vi "TDMS Initialization VI.vi"(8 "error in (no error)":errorcluster, 10 "Custom XML":string, 11 "Device Item Ref in":T1 format="%.0x") -> (0 "error out":errorcluster, 3 "Device Item Ref out":T1 format="%.0x")   [LabVIEW 2011, in "TDMS Custom Device.lvlib"]
uses:
  TDMS Custom Device.lvlib
  <vilib>/NI Veristand/Custom Device API/Custom Device Item Ref.ctl
  <vilib>/NI Veristand/Custom Device API/Custom Device Channel.ctl
  <vilib>/NI Veristand/Custom Device API/Custom Device Channel Type.ctl
  <vilib>/NI Veristand/Custom Device API/Custom Device API.lvlib
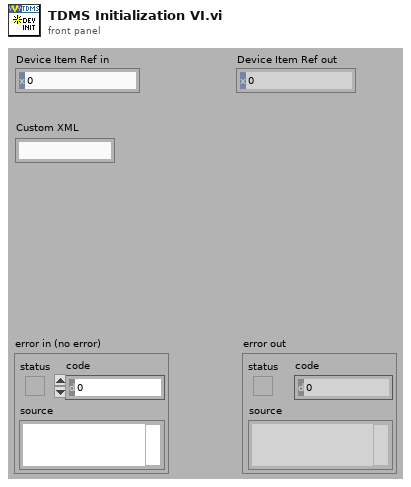
[diagram p1: front panel]
types:
  T1 = typedef "Custom Device API.lvlib/Custom Device Item Ref.ctl" = u64
  T2 = enum16{"Play and Repeat Last", "Stop (and Reset)", "Loop", "Pause"}
  T3 = typedef "Custom Device API.lvlib/Custom Device Channel.ctl" = cluster{"Type":T4, "Units":string, "Default Value":dbl, "Faultable":bool, "Scalable":bool}
  T4 = typedef "Custom Device API.lvlib/Custom Device Channel Type.ctl" = enum16{"Input", "Output"}
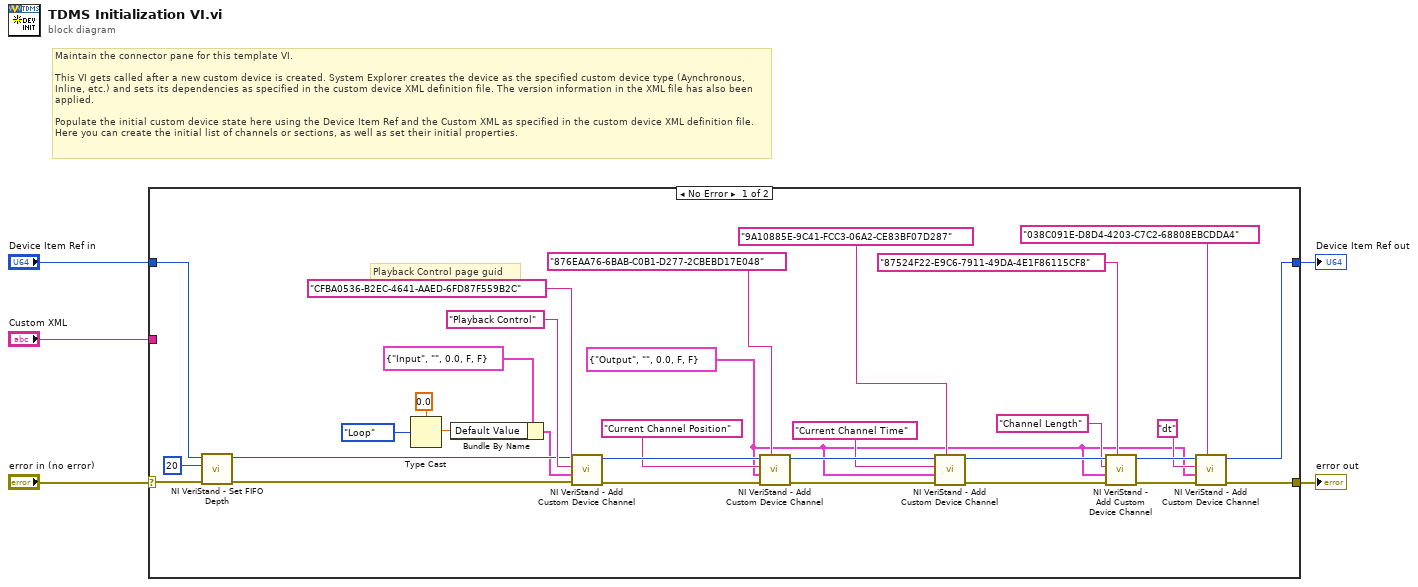
[diagram p0: block diagram]
diagram:
  # "Maintain the connector pane for this template VI.\n\nThis VI gets called after a new custom device is created. System Explorer creates the device as the specified custom device type (Aynchronous, Inline, etc.) and sets its dependencies as specified in the custom device XML definition file. The version information in the XML file has also been applied.\n\nPopulate the initial custom device state here using the Device Item Ref and the Custom XML as specified in the custom device XML definition file. Here you can create the initial list of channels or sections, as well as set their initial properties."
  n1 = case shown="No Error" "error in (no error)" {
    selector: "error in (no error)" -> [w31 w38]
    tunnel: [w19 w38] -> w5
    tunnel: [w18 w37] -> w3
    tunnel: "Device Item Ref in" -> [w32 w37]
    tunnel: "Custom XML" -> [_ _]
    frame No Error {
      w6 = T3 {"Type"=enum."Output", "Units"="", "Default Value"=0.0, "Faultable"=FALSE, "Scalable"=FALSE} ("Channel")
      # "Playback Control page guid"
      n2 = call <vilib>:"NI VeriStand - Set FIFO Depth.vi"("error in (no error)"=w31, "Size FIFO Source (1)"=u32 20, "Device Ref in"=w32) -> ("error out"=w34:errorcluster, "Device Ref out"=w33:T1)  [unwired: 7 in]
      n3 = Type Cast(type=0.0 ("Default Value"), x=T2."Loop" ("Starting mode")) -> (*(type *) &x=w27:dbl)
      n4 = Bundle By Name(cluster=T3 {"Type"=enum."Input", "Units"="", "Default Value"=0.0, "Faultable"=FALSE, "Scalable"=FALSE} ("Channel"), "Default Value"=w27) -> (w25:T3)
      n5 = call <vilib>:"NI VeriStand - Add Custom Device Channel.vi"("GUID (Default Channel)"="CFBA0536-B2EC-4641-AAED-6FD87F559B2C", "error in (no error)"=w34, "Channel"=w25, "Channel Name"="Playback Control", "Parent Ref in"=w33) -> ("error out"=w23:errorcluster, "Parent Ref out"=w24:T1)  [unwired: 3 in, 2 out]
      n6 = call <vilib>:"NI VeriStand - Add Custom Device Channel.vi"("GUID (Default Channel)"="876EAA76-6BAB-C0B1-D277-2CBEBD17E048", "error in (no error)"=w23, "Channel"=w6, "Channel Name"="Current Channel Position", "Parent Ref in"=w24) -> ("error out"=w22:errorcluster, "Parent Ref out"=w15:T1)  [unwired: 3 in, 2 out]
      n7 = call <vilib>:"NI VeriStand - Add Custom Device Channel.vi"("GUID (Default Channel)"="9A10885E-9C41-FCC3-06A2-CE83BF07D287", "error in (no error)"=w22, "Channel"=w6, "Channel Name"="Current Channel Time", "Parent Ref in"=w15) -> ("error out"=w21:errorcluster, "Parent Ref out"=w16:T1)  [unwired: 3 in, 2 out]
      n8 = call <vilib>:"NI VeriStand - Add Custom Device Channel.vi"("GUID (Default Channel)"="87524F22-E9C6-7911-49DA-4E1F86115CF8", "error in (no error)"=w21, "Channel"=w6, "Channel Name"="Channel Length", "Parent Ref in"=w16) -> ("error out"=w20:errorcluster, "Parent Ref out"=w17:T1)  [unwired: 3 in, 2 out]
      n9 = call <vilib>:"NI VeriStand - Add Custom Device Channel.vi"("GUID (Default Channel)"="038C091E-D8D4-4203-C7C2-68808EBCDDA4", "error in (no error)"=w20, "Channel"=w6, "Channel Name"="dt", "Parent Ref in"=w17) -> ("error out"=w19:errorcluster, "Parent Ref out"=w18:T1)  [unwired: 3 in, 2 out]
    }
    frame Error {
    }
  }
  "error out" <- w5
  "Device Item Ref out" <- w3
